vi "Scan Restart.vi"(8 "error in (no error)":errorcluster, 10 "Enable Scan Reset (T: Enable)":bool=TRUE, 11 "VISA resource name":refnum<visa-resource-name>) -> (0 "error out":errorcluster, 3 "VISA resource name out":refnum<visa-resource-name>)   [LabVIEW 2023, in "Keithley DMM6500 DAQ6500 Series.lvlib"]
doc: "Causes a scan to automatically restart if it was interrupted by a power failure."
uses:
  <instrlib>/Keithley DMM6500 DAQ6500 Series/Keithley DMM6500 DAQ6500 Series.lvlib
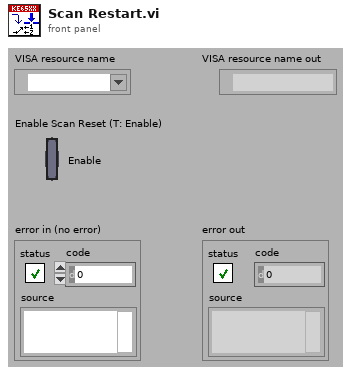
[diagram p1: front panel]
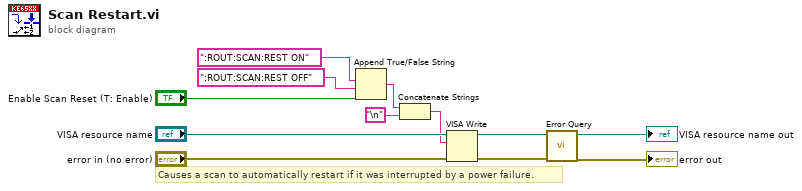
[diagram p0: block diagram]
diagram:
  # "Causes a scan to automatically restart if it was interrupted by a power failure."
  n1 = Append True/False String(1:"Enable Scan Reset (T: Enable)", 2:":ROUT:SCAN:REST OFF", 3:":ROUT:SCAN:REST ON") -> (0:w2:string)  [unwired: 1 in]
  n2 = Concatenate Strings(w2, "\n") -> (w3:string)
  n3 = VISA Write(VISA resource name="VISA resource name", write buffer=w3, error in (no error)="error in (no error)") -> (VISA resource name out=w7:refnum<visa-resource-name>, error out=w6:errorcluster)  [unwired: 1 out]
  n4 = call <instrlib>:"Error Query.vi"("error in (no error)"=w6, "VISA resource name"=w7) -> ("error out"=→"error out":errorcluster, "VISA resource name out"=→"VISA resource name out":refnum<visa-resource-name>)  [unwired: 6 in, 2 out]
